vi "GlobalRect_to_ROI Descriptor.vi"(1 "Global Rectangle":i32[](array[numeric])) -> (0 "ROI Descriptor":T1)   [LabVIEW 2014]
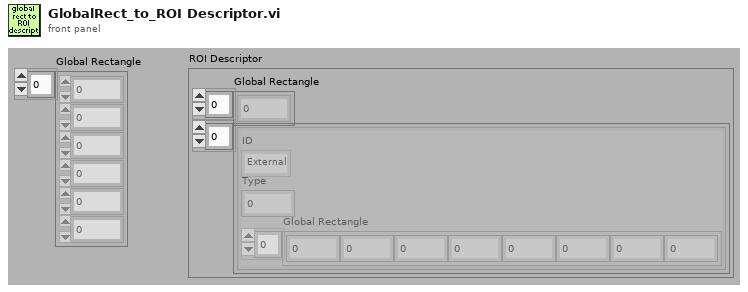
[diagram p1: front panel]
types:
  T1 = cluster{"Global Rectangle":i32[], cluster{"ID":enum32{"External", "Internal"}, "Type":u32, "Global Rectangle":i32[]}[]}
  T2 = cluster{"ID":enum32{"External", "Internal"}, "Type":u32, "Global Rectangle":i32[]}
  T3 = cluster{"ID":enum32{"External", "Internal"}, "Type":u32, "Global Rectangle":i32[]}[]
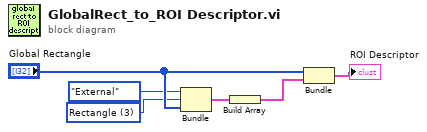
[diagram p0: block diagram]
diagram:
  w2 = u32 3 items=["No Selection", "Point", "Line", "Rectangle", "Oval", "Polygon", "Freehand Region", "Annulus", "Unused2", "Unused3", "Broken Line", "Freehand Line", "Rotated Rectangle"] ("Type")
  n1 = Bundle("ID"=enum32{"External", "Internal"}."External", "Type"=w2, "Global Rectangle"="Global Rectangle") -> (w4:T2)  [unwired: 1 out]
  n2 = Build Array(w4) -> (w5:T3)
  n3 = Bundle("Global Rectangle"="Global Rectangle", w5) -> (→"ROI Descriptor":T1)  [unwired: 1 out]
